vi "Write Linux Desktop.vi"(10 "Linux Desktop":T1={"Username"="plotz", "IP Address"="127.0.0.1", "Path to ts_opensplice source"=path "/home/plotz/lsst_ts/ts_opensplice", "Path to ts_sal source"=path "/home/plotz/lsst_ts/ts_sal"}, 11 "FileTransfer in":refnum<class "FileTransfer.lvclass">) -> (3 "FileTransfer out":refnum<class "FileTransfer.lvclass">)   [LabVIEW 2016, in "FileTransfer.lvclass"]
uses:
  FileTransfer.lvclass
  FileTransfer.lvclass/FileTransfer.ctl
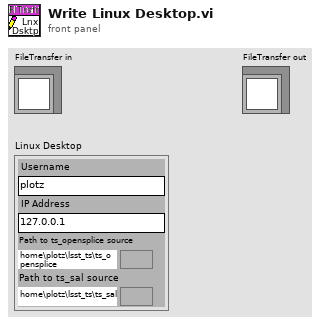
[diagram p1: front panel]
types:
  T1 = cluster{"Username":string, "IP Address":string, "Path to ts_opensplice source":path, "Path to ts_sal source":path}
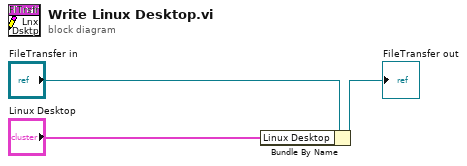
[diagram p0: block diagram]
diagram:
  n1 = Bundle By Name(cluster="FileTransfer in", "Linux Desktop"="Linux Desktop") -> (→"FileTransfer out":refnum<class "FileTransfer.lvclass">)
